vi "Module Type Updated.vi"(8 "error in":errorcluster, 10 "Module Type":T1=enum."Module type: Cloneable") -> (0 "error out":errorcluster)   [LabVIEW 2019, in "Panther Dashboard.lvlib"]
doc: "Module Type Updated\n_____\nCreated using DQMH Event Scripter 6.1.0.128."
uses:
  Panther Dashboard.lvlib
  Module type--enum.ctl
  Module Type Updated Argument--cluster.ctl
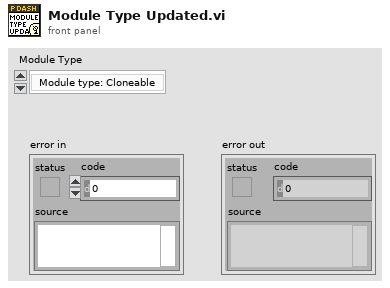
[diagram p1: front panel]
types:
  T1 = typedef "Panther Dashboard.lvlib/Module type--enum.ctl" = enum16{"Module type: Singleton", "Module type: Cloneable"}
  T2 = typedef "Panther Dashboard.lvlib/Module Type Updated Argument--cluster.ctl" = cluster{"Module Type":T1}
  T3 = typedef "Panther Dashboard.lvlib/Broadcast Events--cluster.ctl" = cluster{"Module Did Init":refnum<user-event>, "Status Updated":refnum<user-event>, "Error Reported":refnum<user-event>, "Module Did Stop":refnum<user-event>, "Update Module Execution Status":refnum<user-event>, "References Updated":refnum<user-event>, "Projects Updated":refnum<user-event>, "Targets Updated":refnum<user-event>, "Progress updated":refnum<user-event>, "Scale Updated":refnum<user-event>, "Connector Pane Updated":refnum<user-event>, "Documentation Updated":refnum<user-event>, "Module Type Updated":refnum<user-event>, "Theme Updated":refnum<user-event>, "Project Description Updated":refnum<user-event>}
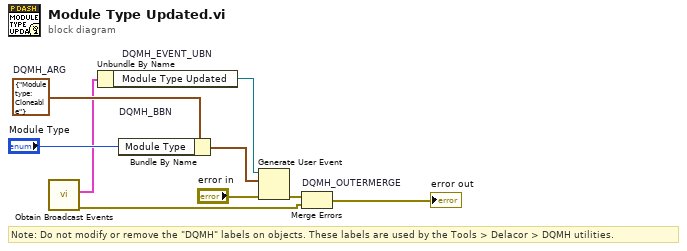
[diagram p0: block diagram]
diagram:
  w4 = T2 {"Module Type"=enum."Module type: Cloneable"}  # DQMH_ARG
  # "Note: Do not modify or remove the \"DQMH\" labels on objects. These labels are used by the Tools > Delacor > DQMH utilities."
  n1 = call "Obtain Broadcast Events.vi"() -> ("error out"=w2:errorcluster, "Panther Dashboard Broadcast Events"=w1:T3)  [unwired: 10 in]
  n2 = Unbundle By Name "DQMH_EVENT_UBN"(w1) -> ("Module Type Updated"=w6:refnum<user-event>)
  n3 = Bundle By Name "DQMH_BBN"(cluster=w4, "Module Type"="Module Type") -> (w7:T2)
  n4 = Generate User Event(user event=w6, event data cluster=w7, error in="error in") -> (error out=w5:errorcluster)  [unwired: 1 in, 1 out]
  n5 = Merge Errors "DQMH_OUTERMERGE"(w5, w2) -> (→"error out":errorcluster)
